vi "Initialize REF Channels.vi"(8 "error in (no error)":errorcluster, 11 "Instrument.DAQ":refnum<class "Instrument.DAQ.lvclass">) -> (0 "error out":errorcluster, 3 "Instrument.DAQ out":refnum<class "Instrument.DAQ.lvclass">)   [LabVIEW 2019, in "Instrument.Lockin.lvlib" / "Instrument.DAQ.lvclass"]
uses:
  Instrument.DAQ.lvclass
  Instrument.DAQ.lvclass/Instrument.DAQ.ctl
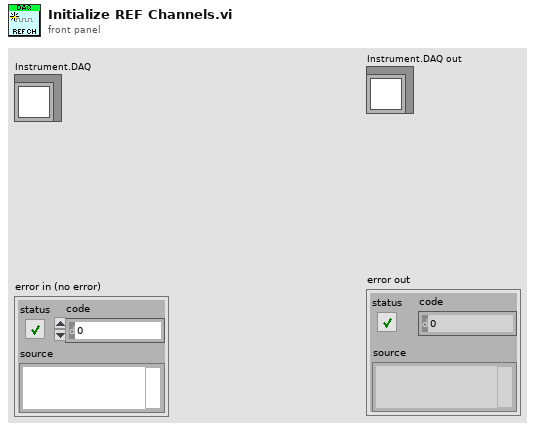
[diagram p1: front panel]
types:
  T1 = typedef "Instrument.Lockin.lvlib/Instrument.DAQ.lvclass/REF.Channel--Cluster--Array.ctl" = T2[]
  T2 = typedef "Instrument.Lockin.lvlib/Instrument.DAQ.lvclass/REF.Channel--Cluster.ctl" = cluster{"Enable?":bool, "Channel":i32, "Frequency":dbl, "Phase":dbl, "TC":dbl, "Roll-Off":i32}
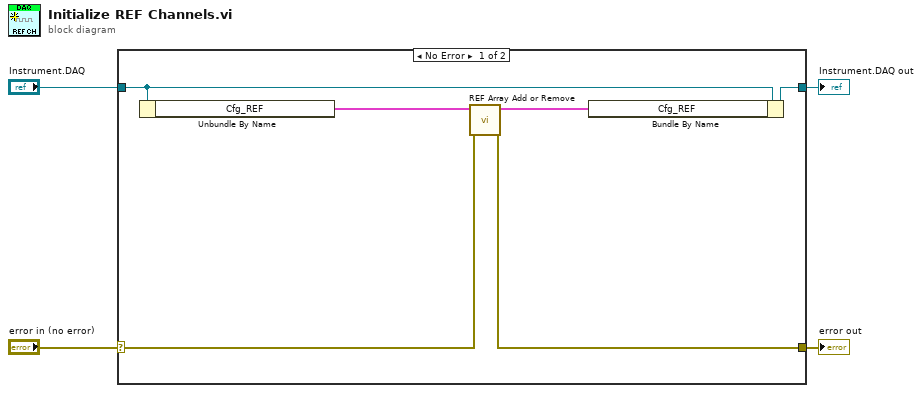
[diagram p0: block diagram]
diagram:
  n1 = case shown="No Error" "error in (no error)" {
    selector: "error in (no error)" -> [w8 w12]
    tunnel: "Instrument.DAQ" -> [w9 w11]
    tunnel: [w10 w11] -> w3
    tunnel: [w7 w12] -> w1
    frame No Error {
      n2 = Unbundle By Name(w9) -> ("Cfg_REF"=w6:T1)
      n3 = call "REF Array Add or Remove.vi"("error in (no error)"=w8, "REF Channels in"=w6) -> ("error out"=w7:errorcluster, "REF Channels out"=w5:T1)  [unwired: 8 in]
      n4 = Bundle By Name(cluster=w9, "Cfg_REF"=w5) -> (w10:refnum<class "Instrument.DAQ.lvclass">)
    }
    frame Error {
    }
  }
  "Instrument.DAQ out" <- w3
  "error out" <- w1
